vi "String to Variant.vi"(8 "error in (no error)":errorcluster, 10 "String":string, 11 "String Value in":refnum<class "String Value.lvclass">) -> (0 "error out":errorcluster, 2 "Variant":variant, 3 "String Value out":refnum<class "String Value.lvclass">)   [LabVIEW 2020, in "Composed Columns.lvlib" / "String Value.lvclass"]
uses:
  String Value.lvclass
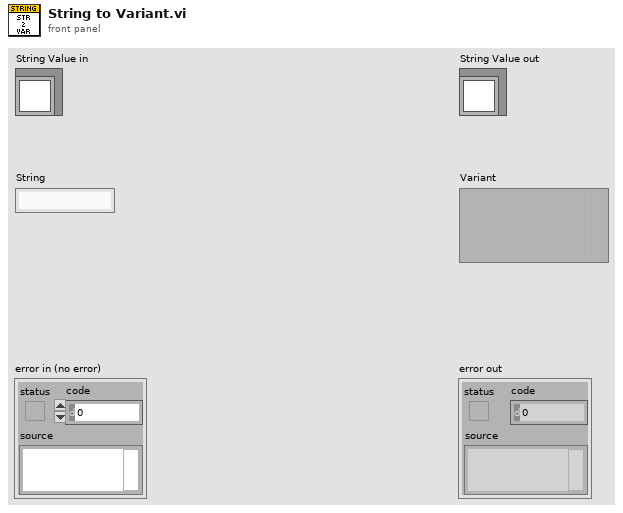
[diagram p1: front panel]
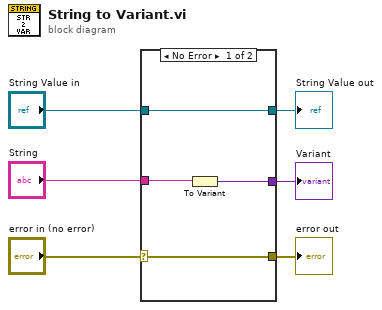
[diagram p0: block diagram]
diagram:
  n1 = case shown="No Error" "error in (no error)" {
    selector: "error in (no error)" -> [w10 w11]
    tunnel: [w10 w11] -> w5
    tunnel: "String Value in" -> [w9 w12]
    tunnel: [w9 w12] -> w3
    tunnel: "String" -> [w8 _]
    tunnel: [w7 _] -> w1
    frame No Error {
      n2 = To Variant(anything=w8) -> (Variant=w7:variant)
    }
    frame Error {
    }
  }
  "error out" <- w5
  "String Value out" <- w3
  "Variant" <- w1
